vi "Configure Frequency.vi"(0 "VISA resource name":refnum<visa-resource-name>, 1 "Aperture (0.1 s)":i32(ring)=1 items=["0.01 s", "0.1 s", "1 s"], 5 "error in (no error)":errorcluster, 6 "Function":i32(ring) items=["Primary", "Secondary"], 8 "Threshold Range":dbl=10.0 min=0.1 max=750.0 format="%#_6p", 9 "Auto  Range (T)":bool=TRUE) -> (14 "VISA resource name out":refnum<visa-resource-name>, 19 "error out":errorcluster)   [LabVIEW 2024, in "Keithley 2100 Series.lvlib"]
doc: "KE2100 uses an on-board counter with 25MHz to measure the frequency (period). The measurement band is from 3Hz to 300kHz (or 333 ms to 3.3 ìs) and the measurement voltages range from 100mV to 750 V in AC. The default for “RANGE” is auto-range."
uses:
  Keithley 2100 Series.lvlib
panel:
  # "Auto"
  # "Custom"
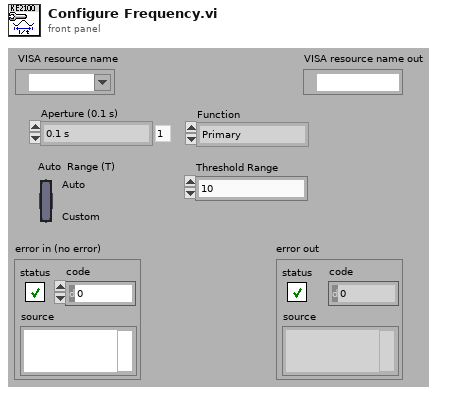
[diagram p1: front panel]
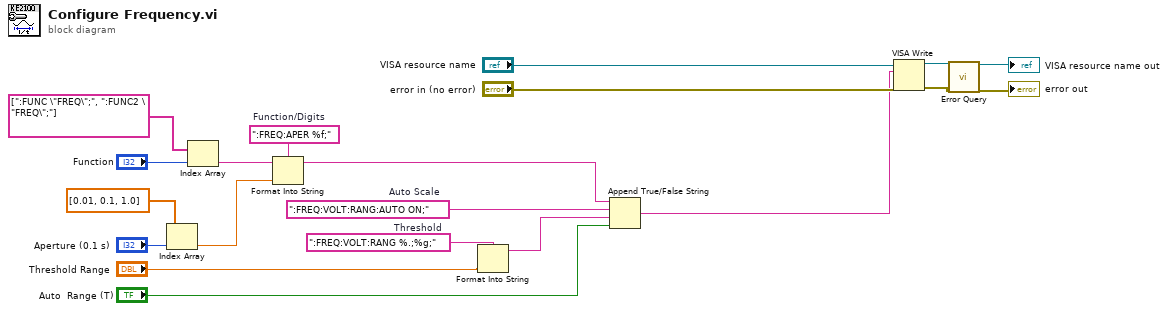
[diagram p0: block diagram]
diagram:
  w1 = ":FREQ:VOLT:RANG:AUTO ON;"  # Auto Scale
  w19 = ":FREQ:VOLT:RANG %.;%g;"  # Threshold
  w20 = ":FREQ:APER %f;"  # Function/Digits
  n1 = Index Array(array=dbl[] [0.01, 0.1, 1.0], index="Aperture (0.1 s)") -> (element=w7:dbl)
  n2 = Index Array(array=string[] [":FUNC \"FREQ\";", ":FUNC2 \"FREQ\";"], index="Function") -> (element=w4:string)
  n3 = Format Into String(format string=w20, initial string=w4, w7) -> (resulting string=w10:string)  [unwired: 1 in, 1 out]
  n4 = Format Into String(format string=w19, "Threshold Range") -> (resulting string=w2:string)  [unwired: 2 in, 1 out]
  n5 = Append True/False String(1:"Auto  Range (T)", 2:w2, 3:w1, 4:w10) -> (0:w9:string)
  n6 = VISA Write(VISA resource name="VISA resource name", write buffer=w9, error in (no error)="error in (no error)") -> (VISA resource name out=w12:refnum<visa-resource-name>, error out=w11:errorcluster)  [unwired: 1 out]
  n7 = call "Error Query.vi"("VISA resource name"=w12, "error in (no error)"=w11) -> ("VISA resource name out"=→"VISA resource name out":refnum<visa-resource-name>, "error out"=→"error out":errorcluster)  [unwired: 14 in, 2 out]
